vi "Global Objects.vi"() -> ()   [LabVIEW 2014]
uses:
  Motors/Motor Typedef.ctl
  <vilib>/Rock Robotics/WPI/MotorControl/WPI_MotorControlDeviceRef.ctl
  <vilib>/Rock Robotics/WPI/MotorControl/WPI_MotorControlType.ctl
  <vilib>/Rock Robotics/SystemInterfaces/Typedef/FPGA_TypedefDigitalModule.ctl
  <vilib>/Rock Robotics/SystemInterfaces/DIO/FPGA_DIOPWMChannel.ctl
  <vilib>/Rock Robotics/WPI/PWM/WPI_PWMDeadband.ctl
  <vilib>/Rock Robotics/WPI/CAN/Jaguar/SubVIs/WPI_CANJaguar_ControlMode.ctl
  <vilib>/Rock Robotics/WPI/CAN/TalonSRX/WPI_CANTalonSRX_APIControlMode.ctl
  <vilib>/Rock Robotics/WPI/PWM/WPI_PWMTransform_ConPane.ctl
  Joystick/Joystick Info.ctl
  <vilib>/Rock Robotics/WPI/Joystick/WPI_JoystickDevRef.ctl
  <vilib>/Rock Robotics/WPI/Joystick/WPI_JoystickDeviceEnum.ctl
  Pneumatics/Shifter.ctl
  <vilib>/Rock Robotics/WPI/Solenoid/WPI_SolenoidDevRef.ctl
  <vilib>/Rock Robotics/WPI/Solenoid/WPI_SolenoidChannel.ctl
  Joystick/Teleop Commands.ctl
  NavX/NaxX Info.ctl
  navX Library v2/TypeDefs/Z900_navX_DeviceTypeDef.ctl
  navX Library v2/TypeDefs/Z900_navX_ProtocolTypeDef.ctl
  navX Library v2/TypeDefs/Z900_navX_NotifyPacketTypeDef.ctl
  navX Library v2/TypeDefs/Z900_navX_ActionTypeDef.ctl
  Configuration/Configuration.ctl
  Encoders/Encoder Info.ctl
  <vilib>/Rock Robotics/WPI/Encoder/WPI_EncoderDevRef.ctl
  <vilib>/Rock Robotics/SystemInterfaces/Encoder/FPGA_EncoderIdx.ctl
  <vilib>/Rock Robotics/SystemInterfaces/Counter/FPGA_CounterCtrSystemIndex.ctl
  <vilib>/Rock Robotics/WPI/Encoder/WPI_EncoderType.ctl
  navX Library v2/navX Library v2.lvlib
panel:
  in  "NavX Zero Point":dbl=-20.58
  out "Right Encoder":T1={"EncoderDevRef"={"DevStatus"={"status"=FALSE, "code"=0, "source"=""}, "EncoderIndex"=enum."Enc 1", "CounterIndex"=enum."Invalid", "DistancePerCount"=0.00436332312, "Decoding Type"=enum."4x"}}
  out "Left Encoder":T1={"EncoderDevRef"={"DevStatus"={"status"=FALSE, "code"=0, "source"=""}, "EncoderIndex"=enum."Enc 0", "CounterIndex"=enum."Invalid", "DistancePerCount"=0.00436332312, "Decoding Type"=enum."4x"}}
  in  "configuration":T6={"Throttle Dead Zone"=0.1, "Throttle Ramp Rate"=0.05, "Turn Dead Zone"=0.1, "Auton"={"Motion Plan P"=0.2, "Motion Plan I"=0.02, "Motion Plan D"=0.05}, "Auto Upshift Enabled"=TRUE, "Upshift Min Throttle"=0.7, "Upshift Min Velocity"=5.0, "Min time before upshift"=500.0, "Shift Throttle Detent"=150, "Min time before downshift"=100.0, "Turn PID"={"Motion Plan P"=0.2, "Motion Plan I"=0.02, "Motion Plan D"=0.05}, "Auto Coast Downshift"=TRUE, "Downshift Coast Max Vel"=10.0, "Downshift Coast Throttle Epsilon"=0.1}
  out "NavX Info":T7={"navX Device"={"Interface"={"Protocol"=enum."SPI", "Update Rate (4Hz-60Hz)"=50, "navX Open TypeDef"=variant(cluster{"SPI Bus":enum16{"SPI On-Board, CS0", "SPI On-Board, CS1", "SPI On-Board, CS2", "SPI On-Board, CS3", "SPI MXP", "Invalid"}, "Clock Rate (Hz)":dbl} {"SPI Bus"=enum."SPI MXP", "Clock Rate (Hz)"=2000000.0})}, "Notify Packet"=refnum, "Loop VI Refnum"=refnum, "Ready to Close Occurrence Refnum"=refnum}, "Current Yaw"=-20.92, "Active"=TRUE} {"navX Device"."Interface"."Update Rate (4Hz-60Hz)" min=4 max=60 step=1}
  in  "Teleop Commands":T10={"Throttle"=-0.0, "Turn"=0.0, "Up Shift Commanded"=FALSE, "Down Shift Commanded"=FALSE}
  out "Shifter":T11={"SolenoidDevRef"={"DevStatus"={"status"=FALSE, "code"=0, "source"=""}, "Pneumatics Control Module"=0, "Forward Solenoid Channel"=enum."Solenoid 0", "Reverse Solenoid Channel"=enum."Solenoid 2"}}
  out "Driver's Controller":T14
  in  "Right Motor":T17={"MotorControlDeviceRef"={"DeviceStatus"={"status"=FALSE, "code"=0, "source"=""}, "Type"=enum."CANTalonSRX", "PWM"={"Controller"=enum."Controller 1", "PWM Channel"=enum."PWM 1", "DeadBand"={"Name"="", "maxPositivePwm"=0, "minPositivePwm"=0, "centerPwm"=0, "maxNegativePwm"=0, "minNegativePwm"=0, "angularRange"=0}}, "CAN"={"Device Number"=3, "Control Mode"=enum."Percent VBus", "Semaphore"=refnum, "Max Vout"=12.0, "TalonSRX Control Mode"=enum."Percent VBus"}, "Invert"=TRUE, "TransformRef"=refnum, "InvTransformRef"=refnum}, "Last Motor Power"=0.0}
  in  "Left Motor":T17={"MotorControlDeviceRef"={"DeviceStatus"={"status"=FALSE, "code"=0, "source"=""}, "Type"=enum."CANTalonSRX", "PWM"={"Controller"=enum."Controller 1", "PWM Channel"=enum."PWM 1", "DeadBand"={"Name"="", "maxPositivePwm"=0, "minPositivePwm"=0, "centerPwm"=0, "maxNegativePwm"=0, "minNegativePwm"=0, "angularRange"=0}}, "CAN"={"Device Number"=1, "Control Mode"=enum."Percent VBus", "Semaphore"=refnum, "Max Vout"=12.0, "TalonSRX Control Mode"=enum."Percent VBus"}, "Invert"=FALSE, "TransformRef"=refnum, "InvTransformRef"=refnum}, "Last Motor Power"=0.0}
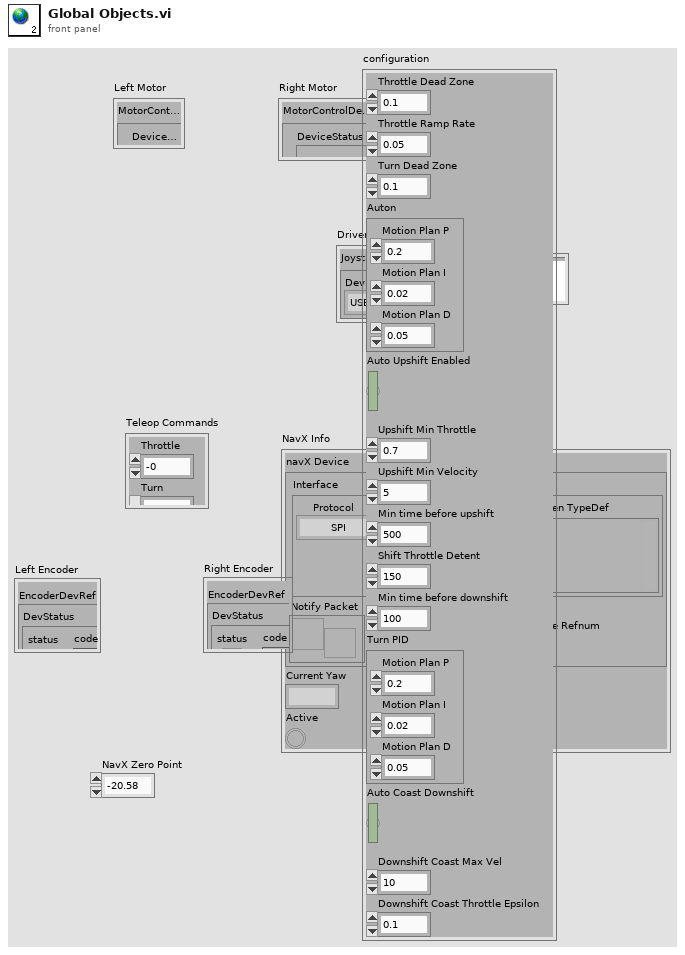
[diagram p1: front panel]
types:
  T1 = typedef "Encoder Info.ctl" = cluster{"EncoderDevRef":T2}
  T2 = typedef "WPI_EncoderDevRef.ctl" = cluster{"DevStatus":errorcluster, "EncoderIndex":T3, "CounterIndex":T4, "DistancePerCount":dbl, "Decoding Type":T5}
  T3 = typedef "FPGA_EncoderIdx.ctl" = enum8{"Enc 0", "Enc 1", "Enc 2", "Enc 3", "Enc 4", "Enc 5", "Enc 6", "Enc 7", "Invalid"}
  T4 = typedef "FPGA_CounterCtrSystemIndex.ctl" = enum8{"Ctr 0", "Ctr 1", "Ctr 2", "Ctr 3", "Ctr 4", "Ctr 5", "Ctr 6", "Ctr 7", "Invalid"}
  T5 = typedef "WPI_EncoderType.ctl" = enum16{"1x", "2x", "4x"}
  T6 = typedef "Configuration.ctl" = cluster{"Throttle Dead Zone":dbl, "Throttle Ramp Rate":dbl, "Turn Dead Zone":dbl, "Auton":cluster{"Motion Plan P":dbl, "Motion Plan I":dbl, "Motion Plan D":dbl}, "Auto Upshift Enabled":bool, "Upshift Min Throttle":dbl, "Upshift Min Velocity":dbl, "Min time before upshift":dbl, "Shift Throttle Detent":u32, "Min time before downshift":dbl, "Turn PID":cluster{"Motion Plan P":dbl, "Motion Plan I":dbl, "Motion Plan D":dbl}, "Auto Coast Downshift":bool, "Downshift Coast Max Vel":dbl, "Downshift Coast Throttle Epsilon":dbl}
  T7 = typedef "NaxX Info.ctl" = cluster{"navX Device":T8, "Current Yaw":dbl, "Active":bool}
  T8 = typedef "navX Library v2.lvlib/Z900_navX_DeviceTypeDef.ctl" = cluster{"Interface":cluster{"Protocol":T9, "Update Rate (4Hz-60Hz)":u8, "navX Open TypeDef":variant}, "Notify Packet":refnum<notifier>, "Loop VI Refnum":refnum<vi>, "Ready to Close Occurrence Refnum":refnum<k4>}
  T9 = typedef "navX Library v2.lvlib/Z900_navX_ProtocolTypeDef.ctl" = enum16{"SERIAL", "I2C", "SPI"}
  T10 = typedef "Teleop Commands.ctl" = cluster{"Throttle":dbl, "Turn":dbl, "Up Shift Commanded":bool, "Down Shift Commanded":bool}
  T11 = typedef "Shifter.ctl" = cluster{"SolenoidDevRef":T12}
  T12 = typedef "WPI_SolenoidDevRef.ctl" = cluster{"DevStatus":errorcluster, "Pneumatics Control Module":u8, "Forward Solenoid Channel":T13, "Reverse Solenoid Channel":T13}
  T13 = typedef "WPI_SolenoidChannel.ctl" = enum8{"Solenoid 0", "Solenoid 1", "Solenoid 2", "Solenoid 3", "Solenoid 4", "Solenoid 5", "Solenoid 6", "Solenoid 7", "Invalid"}
  T14 = typedef "Joystick Info.ctl" = cluster{"JoystickDevRef":T15}
  T15 = typedef "WPI_JoystickDevRef.ctl" = cluster{"Device":T16}
  T16 = typedef "WPI_JoystickDeviceEnum.ctl" = enum16{"USB 0", "USB 1", "USB 2", "USB 3", "USB 4", "USB 5"}
  T17 = typedef "Motor Typedef.ctl" = cluster{"MotorControlDeviceRef":T18, "Last Motor Power":dbl}
  T18 = typedef "WPI_MotorControlDeviceRef.ctl" = cluster{"DeviceStatus":errorcluster, "Type":T19, "PWM":cluster{"Controller":T20, "PWM Channel":T21, "DeadBand":T22}, "CAN":cluster{"Device Number":u8, "Control Mode":T23, "Semaphore":T24, "Max Vout":dbl, "TalonSRX Control Mode":T25}, "Invert":bool, "TransformRef":T26, "InvTransformRef":T26}
  T19 = typedef "WPI_MotorControlType.ctl" = enum16{"PWM", "CAN", "CANTalonSRX"}
  T20 = typedef "FPGA_TypedefDigitalModule.ctl" = enum16{"Controller 1"}
  T21 = typedef "FPGA_DIOPWMChannel.ctl" = enum8{"PWM 0", "PWM 1", "PWM 2", "PWM 3", "PWM 4", "PWM 5", "PWM 6", "PWM 7", "PWM 8", "PWM 9", "PWM MXP 0", "PWM MXP 1", "PWM MXP 2", "PWM MXP 3", "PWM MXP 4", "PWM MXP 5", "PWM MXP 6", "PWM MXP 7", "PWM MXP 8", "PWM MXP 9", "Invalid"}
  T22 = typedef "WPI_PWMDeadband.ctl" = cluster{"Name":string, "maxPositivePwm":i32, "minPositivePwm":i32, "centerPwm":i32, "maxNegativePwm":i32, "minNegativePwm":i32, "angularRange":u16}
  T23 = typedef "WPI_CANJaguar_ControlMode.ctl" = enum8{"Percent VBus", "Current", "Speed", "Position", "Voltage"}
  T24 = typedef "Semaphore RefNum" = refnum<k1>
  T25 = typedef "WPI_CANTalonSRX_APIControlMode.ctl" = enum8{"Percent VBus", "Speed", "Position", "Slave", "Unchanged / Invalid"}
  T26 = typedef "WPI_PWMTransform_ConPane.ctl" = refnum<vi>
diagram:
